vi "Extract Document.vi"(11 "Name":string) -> (2 "Source":string, 3 "Document":string)   [LabVIEW 2020, in "Library Instrument & Equipement.lvlib" / "Library FireBase.lvlib" / "Firebase Driver.lvclass"]
uses:
  Firebase Driver.lvclass
  Firebase Driver.lvclass/Firebase Driver.ctl
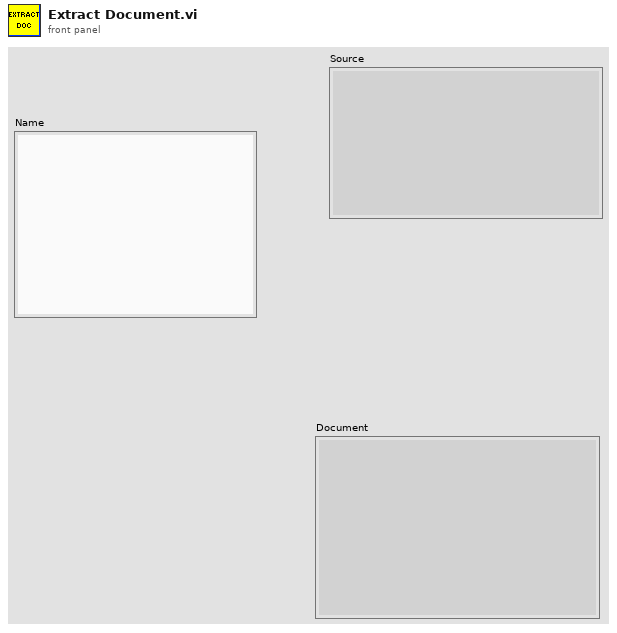
[diagram p1: front panel]
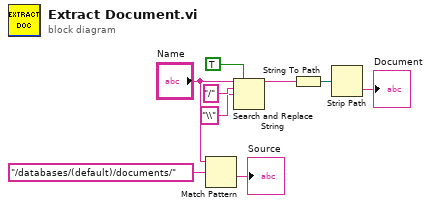
[diagram p0: block diagram]
diagram:
  n1 = Match Pattern(string="Name", regular expression="/databases/(default)/documents/" ("string")) -> (after substring=→"Source":string)  [unwired: 1 in, 3 out]
  n2 = Search and Replace String(replace all?=TRUE ("tout remplacer ? (F)"), input string="Name", search string="/" ("chaîne recherchée"), replace string="\\" ("chaîne de remplacement (\"\")")) -> (result string=w5:string)  [unwired: 4 in, 3 out]
  n3 = String To Path(string=w5) -> (path=w4:path)
  n4 = Strip Path(path=w4) -> (name=→"Document":string)  [unwired: 1 out]
